vi "FromXML.vi"(8 "error in":errorcluster) -> (0 "error out":errorcluster, 3 "TestSuite out":refnum<class "TestSuite.lvclass">)   [LabVIEW 2014, in "TestSuite.lvclass"]
uses:
  TestSuite.lvclass
  TestSuite.lvclass/TestSuite.ctl
  <vilib>/xml/NI_XML.lvlib
  TestCase/TestCase.lvclass
panel:
  in  "TestSuite element":refnum<k20>
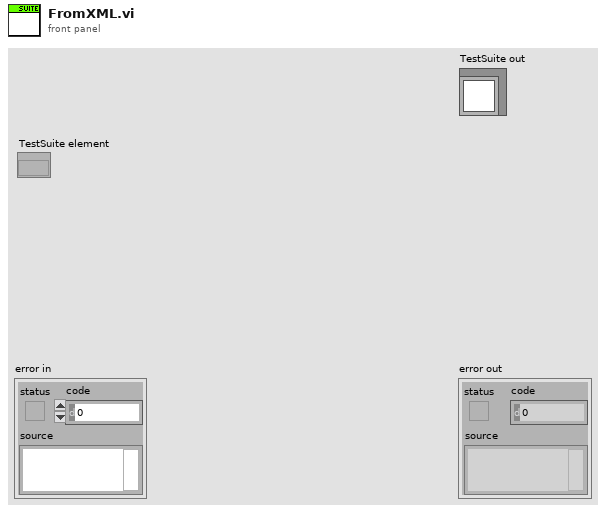
[diagram p1: front panel]
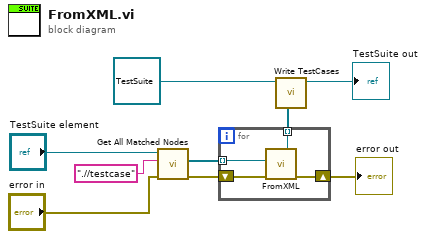
[diagram p0: block diagram]
diagram:
  n1 = call <vilib>:"Get All Matched Nodes.vi"("error in (no error)"="error in", "XPath expression"=".//testcase", "node in"="TestSuite element") -> ("error out"=w5:errorcluster, "node result array"=w4:refnum<k20>[])  [unwired: 6 in, 1 out]
  n2 = for {
    shift-right: [w10] -> w1
    shift-left: w5 -> [w13]
    tunnel: w4 -> [w12] mode=indexing
    tunnel: [w11] -> w3 mode=indexing
    n3 = call "FromXML.vi"("error in"=w13, "TestCase element"=w12) -> ("error out"=w10:errorcluster, "TestCase out"=w11:refnum<class "TestCase.lvclass">)  [unwired: 6 in]
  }
  "error out" <- w1
  n4 = call "Write TestCases.vi"("TestCases"=w3, "TestSuite in"=refnum<class "TestSuite.lvclass"> refnum) -> ("TestSuite out"=→"TestSuite out":refnum<class "TestSuite.lvclass">)  [unwired: 7 in]
